vi "ChannelFlowUNDERGRAD.vi"() -> ()   [LabVIEW 2012]
uses:
  <vilib>/express/express shared/transition.llb/Dynamic To Waveform Array.vi
  <vilib>/express/express shared/transition.llb/Waveform Array To Dynamic.vi
  <vilib>/express/express arith-compare/Formula/Block/exnFormulaBlock how many pts in the wave.vi
  <vilib>/express/express shared/ex_Modify Signal Name.vi
  <vilib>/express/express analysis/Spectral/Block/exnSpectralBlock spectral measurements power poly.vi
  <vilib>/express/express analysis/Spectral/Block/exnSpectralBlock spectral measurements power DDT.vi
  <vilib>/Utility/file.llb/Write To Spreadsheet File (DBL).vi
  <vilib>/express/express arith-compare/Formula/XNode/ExpressFormulaBlockNode.xnode
  <vilib>/express/express analysis/Spectral/XNode/ExpressSpectralMeasurementsBlockNode.xnode
  <vilib>/Analysis/NI_AALBase.lvlib
panel:
  out "Tau(Pa)":dbl
  out "Voltage":dbl
  in  "Samples":i32=40000
  in  "Rate":i32=40000
  out "Waveform Graph":dynamicdata(graph)
  out "Filtered Signal":dynamicdata(graph)
  out "Frequency":dbl
  in  "Zero Voltage":dbl=-3.65209
  out "DC":dbl(knob) scale=0.0..10.0
  out "Delay Elapsed":dbl(slide) caption="Elapsed Time (s)" scale=0.0..1.0
  in  "Freq(Hz) 2":dbl min=0.0 max=60.0 step=1.0 format="%#_3g"
  in  "stop":bool
  in  "Delay Time (s)":dbl=5.0
  in  "Freq Increment":dbl=5.0 min=0.0 max=5.0 step=0.1
  in  "MaxF":dbl=55.0
  out "Flowm (gpm)":dbl
  in  "Freq(Hz)":dbl min=0.0 max=60.0 step=0.1 format="%#_3g"
  out "Waveform Chart":dynamicdata(graph)
  in  "Diaphragm":enum16{"-34", "-20"}(ring)
  out "Time left to save":dbl(slide) scale=0.0..1.0
  in  "Reset Graph":bool caption="Reset"
  out "Moody Diagram":cluster{"Y":dbl[], "Y":dbl[]}[](graph)
  in  "Start of run":dbl
  in  "Write to File?":bool
  in  "OK Button":bool
  in  "Sampling time":dbl=100.0
  in  "Sampling rate\n (0=10Hz)":dbl=100.0
  out "Viscosity (Pa s)":dbl format="%#_6e"
  out "Total Elapsed Time":dbl format="%#.0f"
  in  "stop 2":bool
  out "Bulk Velocity (m/s)":dbl
  in  "File Save Path":path=path "C:/Users/Picasso/Google Drive/Channel Data/SLIPS Data"
  out "Friction Factor":dbl
  out "Reynolds Number":dbl
  out "Density (kg/m^3)":dbl
  in  "Width (m)":dbl=0.1016
  in  "Length (m)":dbl=0.381
  in  "Half-height (m)":dbl=0.00195
  out "Temperature (C)":dbl
  in  "Flow Rate\n (Gpm)":dbl=15.6
  out "Pressure \nDifference (Pa)":dbl
  # "Inputs"
  # "Raw Data"
  # "Calculated Values"
  # "(DO NOT HIT RUN WITH THIS BLANK)"
  # "Pump Settings"
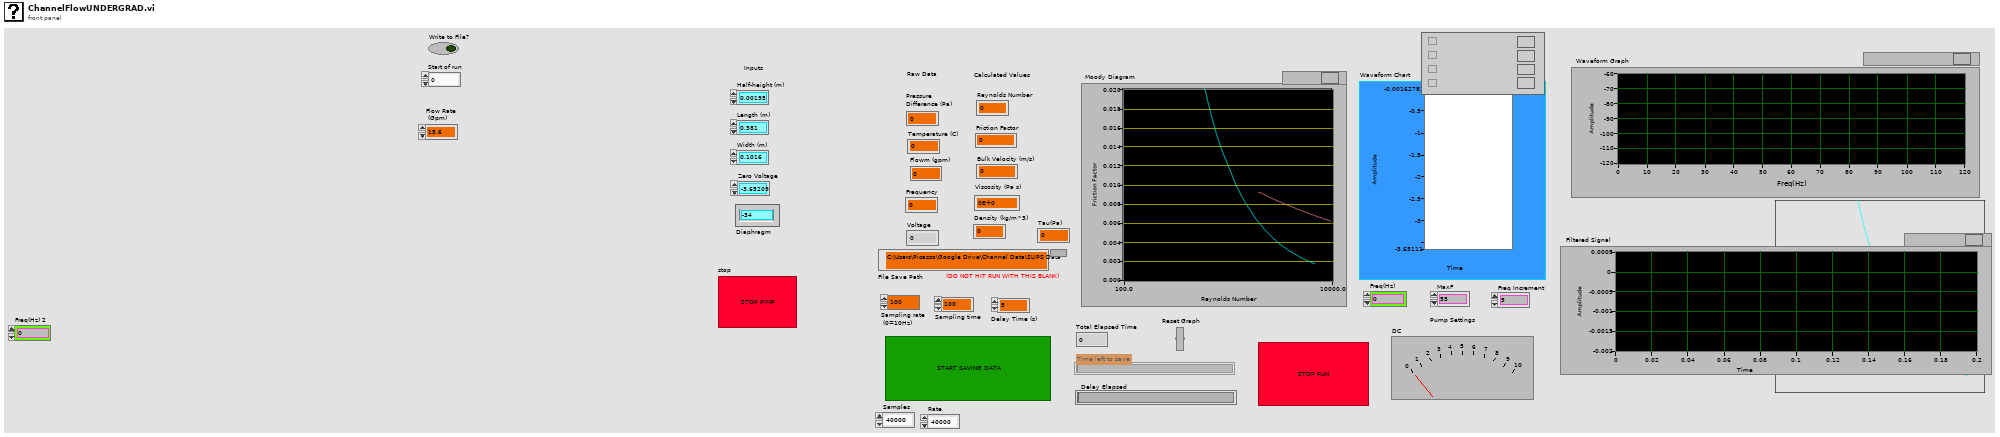
[diagram p1: front panel]
types:
  T1 = cluster{"averaging mode":u16, "weighting mode":u16, "number of averages":u32}
  T2 = cluster{"dB On (F)":bool, "unwrap phase (F)":bool, "convert to degree (F)":bool}
  T3 = enum8{"Enabled", "Disabled", "Disabled and Grayed Out"}
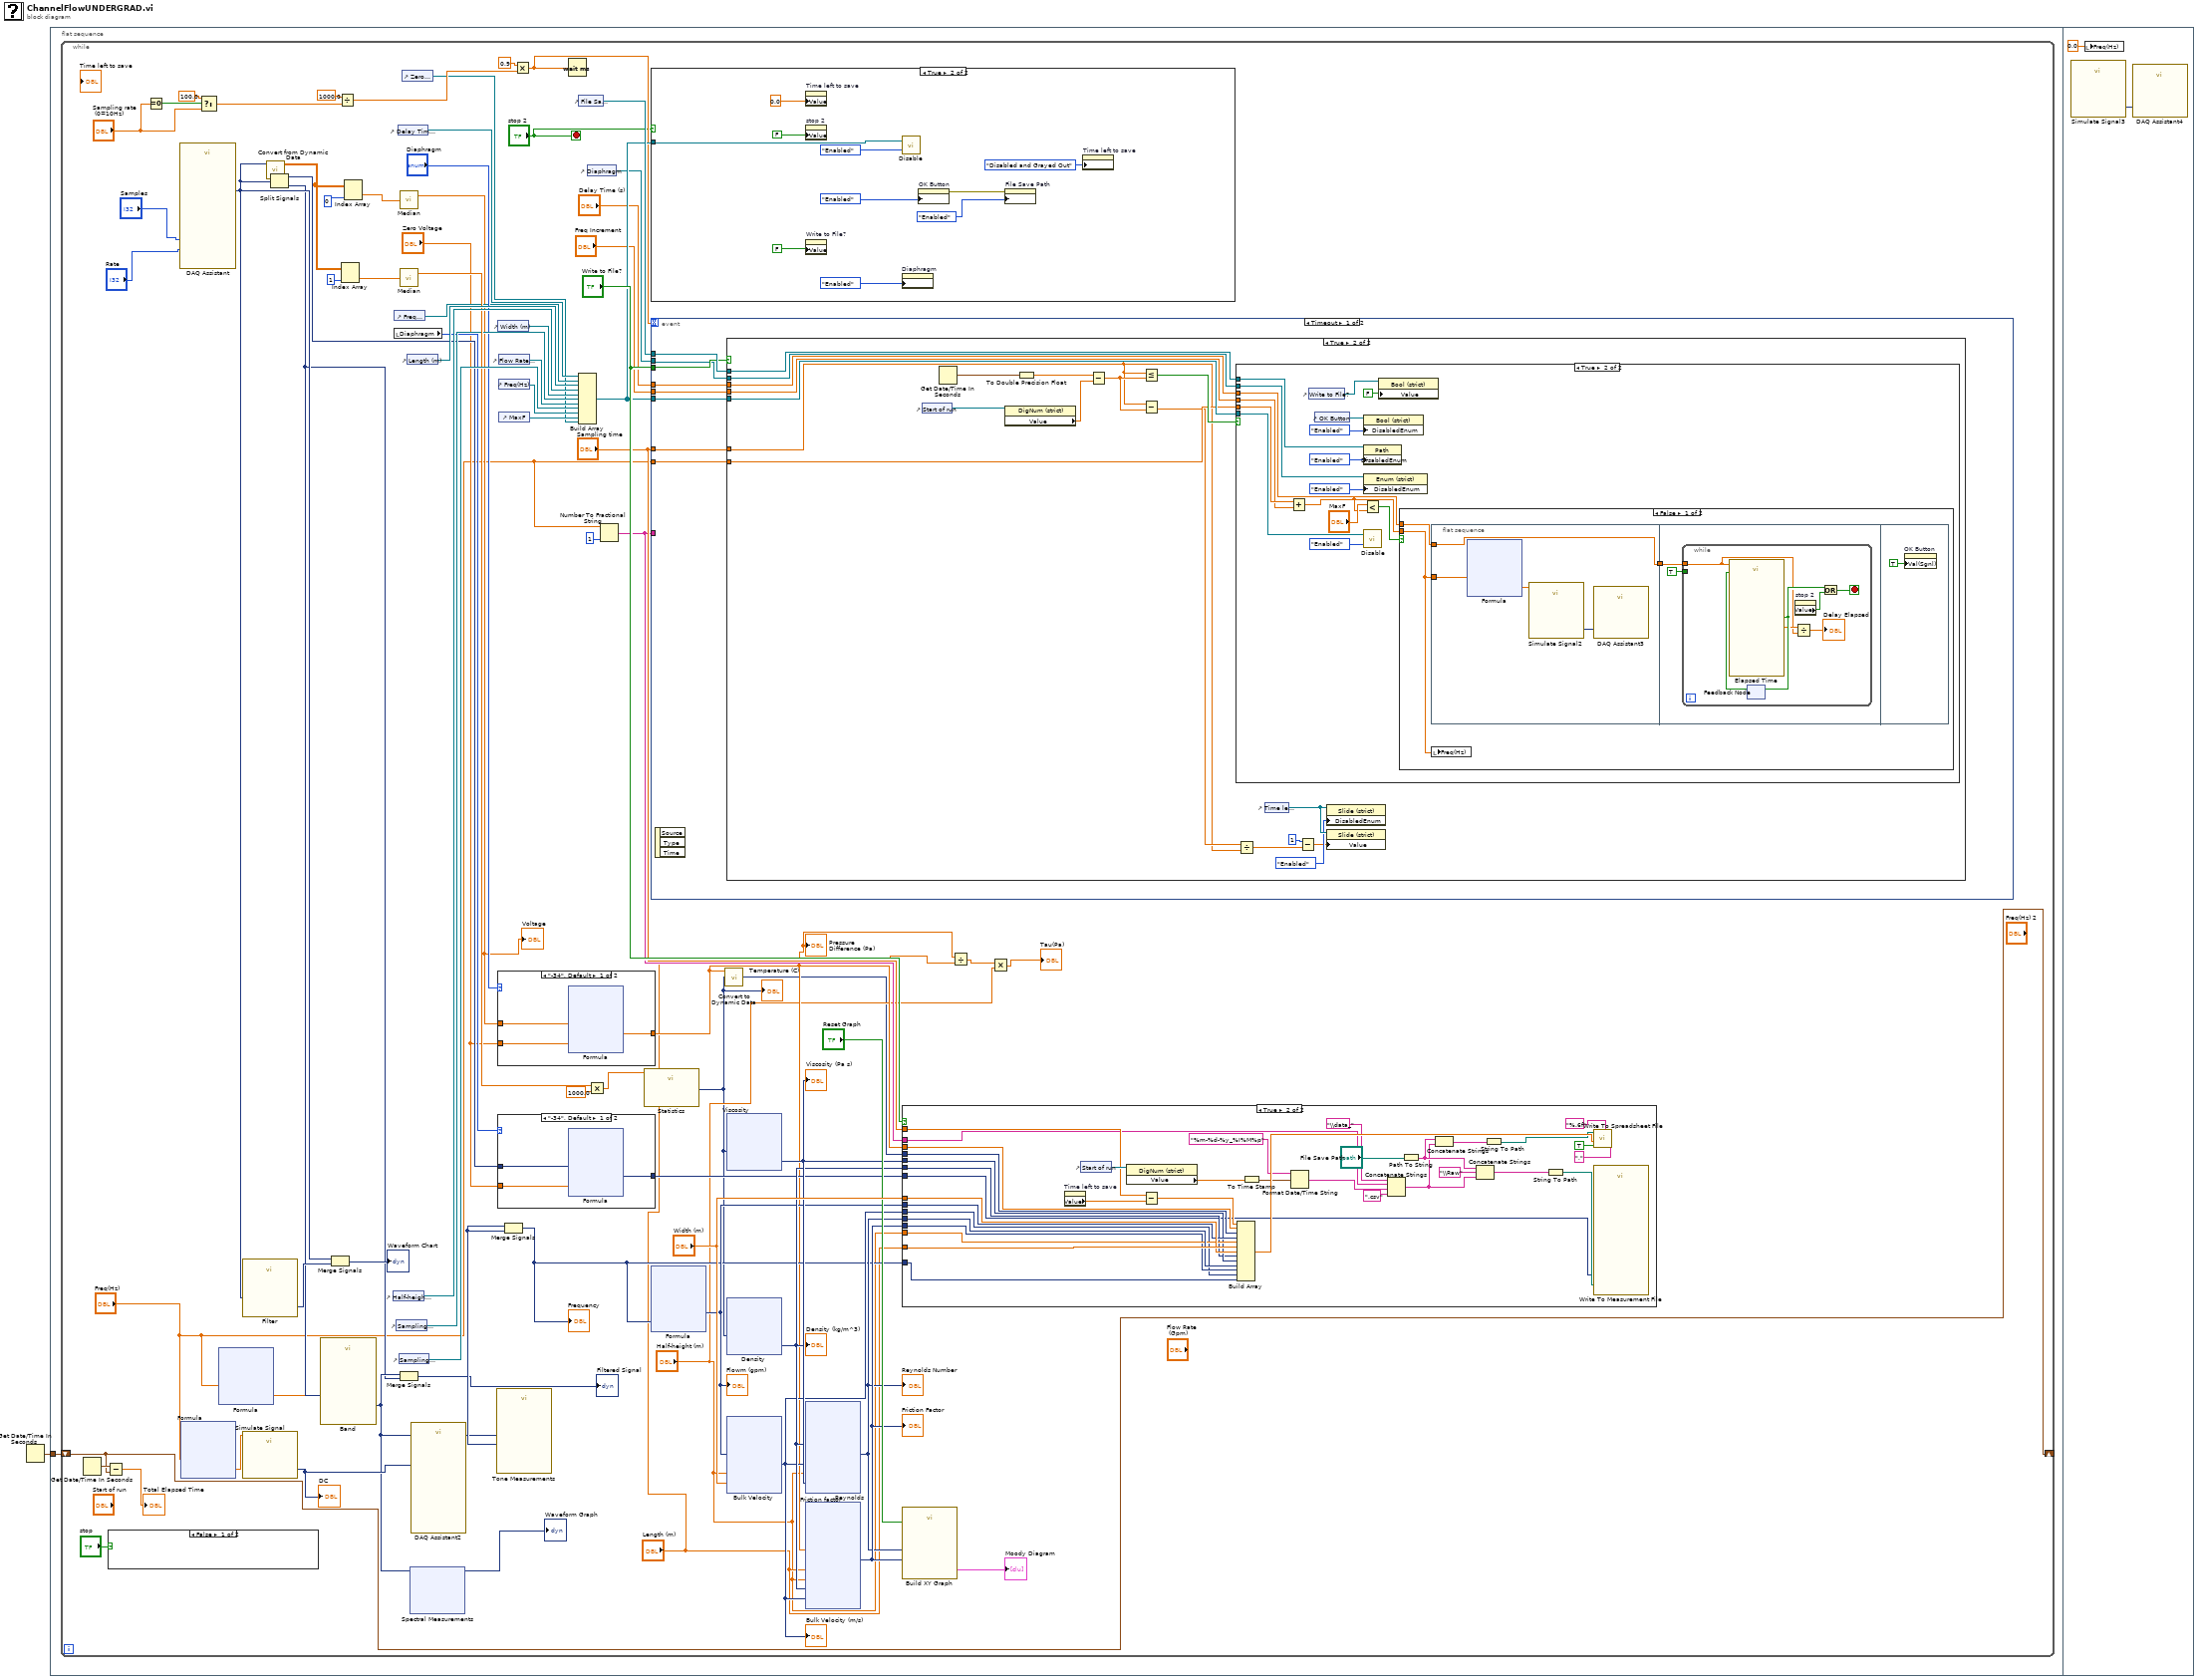
[diagram p0: block diagram]
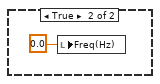
[diagram p2: hidden frame]
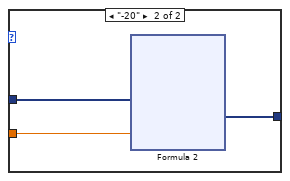
[diagram p3: hidden frame]
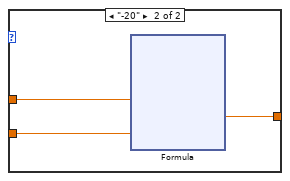
[diagram p4: hidden frame]
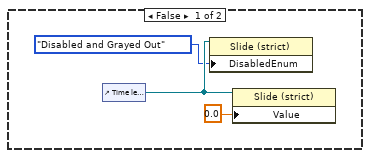
[diagram p7: hidden frame]
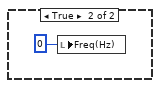
[diagram p9: hidden frame]
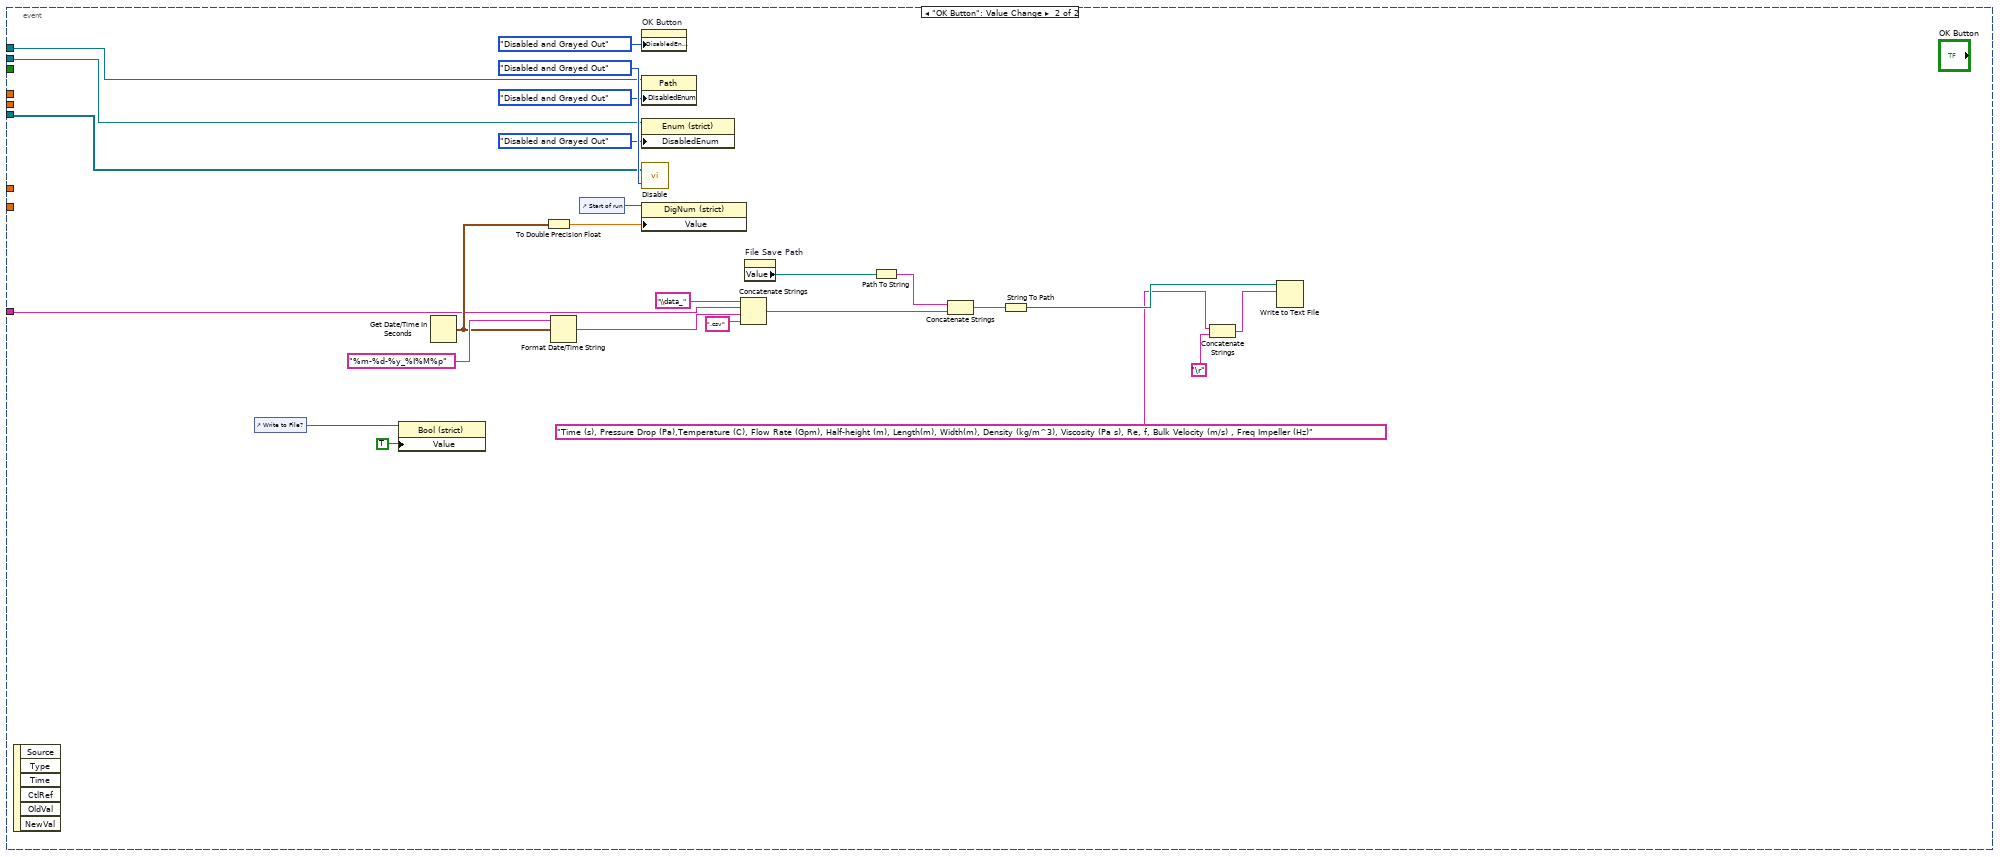
[diagram p10: hidden frame]
diagram:
  n1 = Get Date/Time In Seconds() -> (seconds since 1Jan1904=w1:timestamp)
  n2 = flat-sequence {
    tunnel: w1 -> [w2]
    frame #0 {
      n3 = while {
        shift-right: [w72] -> _
        shift-left: w2 -> [w72]
        stop <- "stop 2" stop-if-true
        n4 = Get Date/Time In Seconds() -> (seconds since 1Jan1904=w73:timestamp)
        n5 = Subtract(x=w73, y=w72) -> (x-y=→"Total Elapsed Time":dbl)
        n6 = case shown="False" "stop" {
          frame False {
          }
          frame True {
            n7 = local write "Freq(Hz)"(0.0) -> ()
          }
        }
        n8 = Equal To 0?(x="Sampling rate\n (0=10Hz)") -> (x = 0?=w69:bool)
        n9 = call "DAQ Assistant"("rate"="Rate", "number of samples"="Samples") -> ("data"=w34:dynamicdata)  [unwired: 15 in, 2 out]
        n10 = xnode "Formula"("X1"="Freq(Hz)") -> ("Result"=w38:dbl)  [unwired: 1 in, 1 out]
        n11 = Select(t=100.0, s=w69, f="Sampling rate\n (0=10Hz)") -> (s? t:f=w68:dbl)
        n12 = xnode "Formula"("X1"="Freq(Hz)") -> ("Result"=w10:dbl)  [unwired: 1 in, 1 out]
        n13 = call "Filter"("Signal"=w34) -> ("Filtered Signal"=w41:dynamicdata)  [unwired: 9 in, 1 out]
        n14 = call "Simulate Signal"("Offset"=w38) -> ("DC"=w37:dynamicdata)  [unwired: 13 in, 1 out]
        "DC" <- w37
        n15 = call "Convert from Dynamic Data"("Dynamic Data Type"=w34) -> ("Array"=w35:dbl[][])  [unwired: 3 in]
        n16 = Split Signals(w34) -> (w25:dynamicdata, w16:dynamicdata)  [unwired: 3 in, 1 out]
        n17 = call "Band"("Lower Cut-Off"=w10, "Signal"=w16) -> ("Filtered Signal"=w19:dynamicdata)  [unwired: 8 in, 1 out]
        n18 = Merge Signals(w34, w41) -> (→"Waveform Chart":dynamicdata)
        n19 = Divide(x=1000.0, y=w68) -> (x/y=w46:dbl)
        n20 = Index Array(array=w35, index (col)=1 ("index")) -> (element=w56:dbl[])  [unwired: 1 in]
        n21 = Index Array(array=w35, index (col)=0 ("index")) -> (element=w55:dbl[])  [unwired: 1 in]
        n22 = control-ref of="Half-height (m)"() -> (w79:refnum<vi>)
        n23 = control-ref of="Freq Increment"() -> (w29:refnum<vi>)
        n24 = local read "Diaphragm"() -> (w26:enum16{"-34", "-20"})
        n25 = control-ref of="Sampling time"() -> (w51:refnum<vi>)
        n26 = control-ref of="Delay Time (s)"() -> (w28:refnum<vi>)
        n27 = control-ref of="Sampling rate\n (0=10Hz)"() -> (w76:refnum<vi>)
        n28 = call <vilib>:"Median.vi"("X"=w55) -> ("median"=w12:dbl)  [unwired: 1 out]
        "Voltage" <- w12
        n29 = call <vilib>:"Median.vi"("X"=w56) -> ("median"=w53:dbl)  [unwired: 1 out]
        n30 = Merge Signals(w19, w16) -> (→"Filtered Signal":dynamicdata)
        n31 = control-ref of="Zero Voltage"() -> (w22:refnum<vi>)
        n32 = control-ref of="Length (m)"() -> (w78:refnum<vi>)
        n33 = xnode "Spectral Measurements"("Signals"=w19) -> ("Power Spectrum"=→"Waveform Graph":dynamicdata)  [unwired: 1 in, 1 out]
        n34 = call "DAQ Assistant2"("data"=w37) -> ()  [unwired: 17 in, 2 out]
        n35 = call "Tone Measurements"("Signals"=w19) -> ("Frequency"=w20:dynamicdata)  [unwired: 9 in, 1 out]
        n36 = control-ref of="Width (m)"() -> (w77:refnum<vi>)
        n37 = case shown="\"-34\", Default" "Diaphragm" {
          tunnel: w12 -> [w531 w544]
          tunnel: [w530 w543] -> w9
          tunnel: "Zero Voltage" -> [w529 w542]
          frame "-34", Default {
            n38 = xnode "Formula"("V"=w531, "X2"=w529) -> ("Result"=w530:dbl)  [unwired: 1 in, 1 out]
          }
          frame "-20" {
            n39 = xnode "Formula"("V"=w544, "X2"=w542) -> ("Result"=w543:dbl)  [unwired: 1 in, 1 out]
          }
        }
        "Pressure \nDifference (Pa)" <- w9
        n40 = case shown="\"-34\", Default" w26 {
          tunnel: [w100 w242] -> w27
          tunnel: w25 -> [w99 w241]
          tunnel: "Zero Voltage" -> [w98 w240]
          frame "-34", Default {
            n41 = xnode "Formula"("V"=w99, "X2"=w98) -> ("Result"=w100:dynamicdata)  [unwired: 1 in, 1 out]
          }
          frame "-20" {
            n42 = xnode "Formula 2"("V"=w241, "X2"=w240) -> ("Result"=w242:dynamicdata)  [unwired: 1 in, 1 out]
          }
        }
        n43 = control-ref of="Flow Rate\n (Gpm)"() -> (w50:refnum<vi>)
        n44 = control-ref of="Freq(Hz)"() -> (w36:refnum<vi>)
        n45 = control-ref of="MaxF"() -> (w32:refnum<vi>)
        n46 = Merge Signals(w20, w20) -> (w15:dynamicdata)
        "Frequency" <- w15
        n47 = Multiply(x=0.9, y=w46) -> (x*y=w43:dbl)
        n48 = Wait (ms)(milliseconds to wait=w43) -> ()  [unwired: 1 out]
        n49 = control-ref of="File Save Path"() -> (w75:refnum<vi>)
        n50 = Build Array(w28, w29, w78, w79, w77, w51, w50, w76, w36, w32, w22) -> (w62:refnum<vi>[])
        n51 = control-ref of="Diaphragm"() -> (w47:refnum<vi>)
        n52 = Multiply(x=w53, y=1000.0) -> (x*y=w4:dbl)
        n53 = Number To Fractional String(number="Freq(Hz)", precision (6)=1) -> (F-format string=w39:string)  [unwired: 2 in]
        n54 = call "Statistics"("Signals"=w4) -> ("Median"=w3:dynamicdata)  [unwired: 25 in, 1 out]
        "Temperature (C)" <- w3
        n55 = case shown="True" "stop 2" {
          tunnel: w62 -> [_ w842]
          frame False {
          }
          frame True {
            n56 = property on="Time left to save" class="Slide (strict)"("Value"=0.0 ("Time left to save")) -> ()  [unwired: 2 in, 2 out]
            n57 = property on="stop 2" class="Bool (strict)"("Value"=FALSE) -> ()  [unwired: 2 in, 2 out]
            n58 = property on="Write to File?" class="Bool (strict)"("Value"=FALSE ("Write to File?")) -> ()  [unwired: 2 in, 2 out]
            n59 = call "Disable.vi"("Disabled"=T3."Enabled", "Array"=w842) -> ()  [unwired: 1 in]
            n60 = property on="Diaphragm" class="Enum (strict)"("DisabledEnum"=T3."Enabled" ("Disabled")) -> ()  [unwired: 2 in, 2 out]
            n61 = property on="OK Button" class="Bool (strict)"("DisabledEnum"=T3."Enabled" ("Disabled")) -> (error out=w839:errorcluster)  [unwired: 2 in, 1 out]
            n62 = property on="File Save Path" class="Path"(error in=w839, "DisabledEnum"=T3."Enabled" ("Disabled")) -> ()  [unwired: 1 in, 2 out]
            n63 = property on="Time left to save" class="Slide (strict)"("DisabledEnum"=T3."Disabled and Grayed Out" ("Disabled")) -> ()  [unwired: 2 in, 2 out]
          }
        }
        n64 = event shown="[0] Timeout" {
          selector: _ -> [_ _]
          dyn-events: _ -> [_ _]
          timeout: w43 -> [_ _]
          tunnel: w62 -> [w1302 w1389]
          tunnel: w75 -> [w1301 w1388]
          tunnel: "Sampling time" -> [w1303 _]
          tunnel: "Write to File?" -> [w1300 _]
          tunnel: w47 -> [w1299 w1374]
          tunnel: w39 -> [_ w1371]
          tunnel: "Freq(Hz)" -> [w1298 _]
          tunnel: "Freq Increment" -> [w1297 _]
          tunnel: "Delay Time (s)" -> [w1296 _]
          event Timeout {
            n65 = event-data() -> ()  [unwired: 1 in, 3 out]
            n66 = case shown="True" w1300 {
              tunnel: w1303 -> [_ w1310]
              tunnel: w1302 -> [_ w1323]
              tunnel: w1301 -> [_ w1322]
              tunnel: w1299 -> [_ w1318]
              tunnel: w1298 -> [_ w1314]
              tunnel: w1297 -> [_ w1313]
              tunnel: w1296 -> [_ w1312]
              frame False {
                n67 = control-ref of="Time left to save"() -> (w1305:refnum<vi>)
                n68 = property class="Slide (strict)"(reference=w1305, "DisabledEnum"=T3."Disabled and Grayed Out" ("Disabled")) -> ()  [unwired: 1 in, 2 out]
                n69 = property class="Slide (strict)"(reference=w1305, "Value"=0.0) -> ()  [unwired: 1 in, 2 out]
              }
              frame True {
                n70 = control-ref of="Start of run"() -> (w1325:refnum<vi>)
                n71 = Get Date/Time In Seconds() -> (seconds since 1Jan1904=w1316:timestamp)
                n72 = property class="DigNum (strict)"(reference=w1325) -> ("Value"=w1324:dbl)  [unwired: 1 in, 2 out]
                n73 = To Double Precision Float(number=w1316) -> (double precision float=w1315:dbl)
                n74 = Subtract(x=w1315, y=w1324) -> (x-y=w1317:dbl)
                n75 = Less Or Equal?(x=w1310, y=w1317) -> (x <= y?=w1321:bool)
                n76 = Subtract(x=w1310, y=w1317) -> (x-y=w1311:dbl)
                n77 = case shown="True" w1321 {
                  tunnel: w1323 -> [_ w1338]
                  tunnel: w1322 -> [_ w1337]
                  tunnel: w1318 -> [_ w1332]
                  tunnel: w1314 -> [_ w1329]
                  tunnel: w1313 -> [_ w1327]
                  tunnel: w1312 -> [_ w1326]
                  frame False {
                  }
                  frame True {
                    n78 = Add(x=w1329, y=w1327) -> (x+y=w1328:dbl)
                    n79 = control-ref of="Write to File?"() -> (w1335:refnum<vi>)
                    n80 = control-ref of="OK Button"() -> (w1336:refnum<vi>)
                    n81 = property class="Bool (strict)"(reference=w1336, "DisabledEnum"=T3."Enabled" ("Disabled")) -> ()  [unwired: 1 in, 2 out]
                    n82 = property class="Path"(reference=w1337, "DisabledEnum"=T3."Enabled" ("Disabled")) -> ()  [unwired: 1 in, 2 out]
                    n83 = property class="Enum (strict)"(reference=w1332, "DisabledEnum"=T3."Enabled" ("Disabled")) -> ()  [unwired: 1 in, 2 out]
                    n84 = Less?(x="MaxF", y=w1328) -> (x < y?=w1330:bool)
                    n85 = call "Disable.vi"("Disabled"=T3."Enabled", "Array"=w1338) -> ()  [unwired: 1 in]
                    n86 = property class="Bool (strict)"(reference=w1335, "Value"=FALSE) -> ()  [unwired: 1 in, 2 out]
                    n87 = case shown="False" w1330 {
                      tunnel: w1328 -> [w1344 _]
                      tunnel: w1326 -> [w1343 _]
                      frame False {
                        n88 = flat-sequence {
                          tunnel: w1344 -> [w1346]
                          tunnel: w1343 -> [w1345]
                          tunnel: [w1345] -> w1342
                          tunnel: w1342 -> [w1358]
                          frame #0 {
                            n89 = xnode "Formula"("X1"=w1346) -> ("Result"=w1348:dbl)  [unwired: 1 in, 1 out]
                            n90 = call "Simulate Signal2"("Offset"=w1348) -> ("DC"=w1347:dynamicdata)  [unwired: 13 in, 1 out]
                            n91 = call "DAQ Assistant3"("data"=w1347) -> ()  [unwired: 17 in, 2 out]
                          }
                          frame #1 {
                            n92 = while {
                              tunnel: w1358 -> [w1360]
                              tunnel: TRUE -> [_]
                              stop <- w1362 stop-if-true
                              n93 = feedback #1() -> (w1365:bool)  [unwired: 1 in]
                              n94 = call "Elapsed Time"("Time Target (s)"=w1360, "Reset"=w1365) -> ("Elapsed Time (s)"=w1361:dbl, "Time has Elapsed"=w1363:bool)  [unwired: 10 in, 6 out]
                              n95 = feedback-in #1(w1363) -> ()
                              n96 = property on="stop 2" class="Bool (strict)"() -> ("Value"=w1364:bool)  [unwired: 2 in, 2 out]
                              n97 = Divide(x=w1361, y=w1360) -> (x/y=→"Delay Elapsed":dbl)
                              n98 = Or(x=w1363, y=w1364) -> (x .or. y?=w1362:bool)
                            }
                          }
                          frame #2 {
                            n99 = property on="OK Button" class="Bool (strict)"("Val(Sgnl)"=TRUE) -> ()  [unwired: 2 in, 2 out]
                          }
                        }
                        n100 = local write "Freq(Hz)"(w1344) -> ()
                      }
                      frame True {
                        n101 = local write "Freq(Hz)"(0) -> ()
                      }
                    }
                  }
                }
                n102 = Divide(x=w1311, y=w1310) -> (x/y=w1309:dbl)
                n103 = control-ref of="Time left to save"() -> (w1320:refnum<vi>)
                n104 = Subtract(x=1, y=w1309) -> (x-y=w1307:dbl)
                n105 = property class="Slide (strict)"(reference=w1320, "DisabledEnum"=T3."Enabled" ("Disabled")) -> ()  [unwired: 1 in, 2 out]
                n106 = property class="Slide (strict)"(reference=w1320, "Value"=w1307) -> ()  [unwired: 1 in, 2 out]
              }
            }
          }
          event "OK Button": Value Change {
            n107 = event-data() -> ()  [unwired: 1 in, 6 out]
            n108 = control-ref of="Write to File?"() -> (w1387:refnum<vi>)
            n109 = property class="Bool (strict)"(reference=w1387, "Value"=TRUE) -> ()  [unwired: 1 in, 2 out]
            n110 = Get Date/Time In Seconds() -> (seconds since 1Jan1904=w1377:timestamp)
            n111 = To Double Precision Float(number=w1377) -> (double precision float=w1384:dbl)
            n112 = Format Date/Time String(time format string (%c)="%m-%d-%y_%I%M%p", seconds (now)=w1377) -> (date/time string=w1372:string)  [unwired: 1 in]
            n113 = control-ref of="Start of run"() -> (w1385:refnum<vi>)
            n114 = property on="OK Button" class="Bool (strict)"("DisabledEnum"=T3."Disabled and Grayed Out" ("Disabled")) -> ()  [unwired: 2 in, 2 out]
            n115 = property class="Path"(reference=w1388, "DisabledEnum"=T3."Disabled and Grayed Out" ("Disabled")) -> ()  [unwired: 1 in, 2 out]
            n116 = property class="Enum (strict)"(reference=w1374, "DisabledEnum"=T3."Disabled and Grayed Out" ("Disabled")) -> ()  [unwired: 1 in, 2 out]
            n117 = call "Disable.vi"("Disabled"=T3."Disabled and Grayed Out", "Array"=w1389) -> ()  [unwired: 1 in]
            n118 = property class="DigNum (strict)"(reference=w1385, "Value"=w1384) -> ()  [unwired: 1 in, 2 out]
            n119 = Concatenate Strings("\\data_", w1371, w1372, ".csv" ("string")) -> (w1379:string)
            n120 = property on="File Save Path" class="Path"() -> ("Value"=w1378:path)  [unwired: 2 in, 2 out]
            n121 = Path To String(path=w1378) -> (string=w1380:string)
            n122 = Concatenate Strings(w1380, w1379) -> (w1381:string)
            n123 = String To Path(string=w1381) -> (path=w1376:path)
            n124 = Concatenate Strings("Time (s), Pressure Drop (Pa),Temperature (C), Flow Rate (Gpm), Half-height (m), Length(m), Width(m), Density (kg/m^3), Viscosity (Pa s), Re, f, Bulk Velocity (m/s) , Freq Impeller (Hz)" ("text"), "\r") -> (w1368:string)
            n125 = Write to Text File(file (use dialog)=w1376, text=w1368) -> ()  [unwired: 2 in, 3 out]
          }
        }
        n126 = xnode "Formula"("X1"=w15) -> ("Result"=w23:dynamicdata)  [unwired: 1 in, 1 out]
        "Flowm (gpm)" <- w23
        n127 = call "Convert to Dynamic Data"("Double"=w9) -> ()  [unwired: 3 in, 1 out]
        n128 = xnode "Viscosity"("T"=w3) -> ("Result"=w60:dynamicdata)  [unwired: 1 in, 1 out]
        "Viscosity (Pa s)" <- w60
        n129 = xnode "Density"("T"=w3) -> ("Result"=w59:dynamicdata)  [unwired: 1 in, 1 out]
        "Density (kg/m^3)" <- w59
        n130 = xnode "Bulk Velocity"("Q"=w23, "h"="Half-height (m)", "w"="Width (m)") -> ("Result"=w49:dynamicdata)  [unwired: 1 in, 1 out]
        "Bulk Velocity (m/s)" <- w49
        n131 = xnode "Reynolds"("r"=w59, "U"=w49, "h"="Half-height (m)", "m"=w60) -> ("Result"=w52:dynamicdata)  [unwired: 1 in, 1 out]
        "Reynolds Number" <- w52
        n132 = xnode "Friction factor"("P"=w9, "L"="Length (m)", "h"="Half-height (m)", "r"=w59, "U"=w49) -> ("Result"=w61:dynamicdata)  [unwired: 1 in, 1 out]
        "Friction Factor" <- w61
        n133 = case shown="True" "Write to File?" {
          tunnel: w23 -> [_ w872]
          tunnel: "Half-height (m)" -> [_ w865]
          tunnel: "Length (m)" -> [_ w878]
          tunnel: "Width (m)" -> [_ w877]
          tunnel: w52 -> [_ w876]
          tunnel: w61 -> [_ w864]
          tunnel: w60 -> [_ w863]
          tunnel: w59 -> [_ w862]
          tunnel: w9 -> [_ w860]
          tunnel: w3 -> [_ w859]
          tunnel: w49 -> [_ w858]
          tunnel: "Sampling time" -> [_ w854]
          tunnel: w39 -> [_ w851]
          tunnel: w27 -> [_ w844]
          tunnel: w15 -> [_ w843]
          frame False {
          }
          frame True {
            n134 = property on="Time left to save" class="Slide (strict)"() -> ("Value"=w856:dbl)  [unwired: 2 in, 2 out]
            n135 = control-ref of="Start of run"() -> (w870:refnum<vi>)
            n136 = property class="DigNum (strict)"(reference=w870) -> ("Value"=w869:dbl)  [unwired: 1 in, 2 out]
            n137 = Subtract(x=w854, y=w856) -> (x-y=w855:dbl)
            n138 = Build Array(w855, w860, w859, w872, w865, w878, w877, w862, w863, w876, w864, w858, w843) -> (w875:dbl[])
            n139 = To Time Stamp(1:w869) -> (0:w868:timestamp)
            n140 = Format Date/Time String(time format string (%c)="%m-%d-%y_%I%M%p", seconds (now)=w868) -> (date/time string=w852:string)  [unwired: 1 in]
            n141 = Concatenate Strings("\\data_", w851, w852, ".csv" ("string")) -> (w845:string)
            n142 = Path To String(path="File Save Path") -> (string=w846:string)
            n143 = Concatenate Strings(w846, w845) -> (w848:string)
            n144 = Concatenate Strings(w846, "\\Raw", w845) -> (w850:string)
            n145 = String To Path(string=w848) -> (path=w866:path)
            n146 = String To Path(string=w850) -> (path=w849:path)
            n147 = call-poly <vilib>:"Write To Spreadsheet File.vi"("delimiter (\\t)"="," ("delimiter (\\t)"), "format (%.3f)"="%.6f", "append to file? (new file:F)"=TRUE, "1D data"=w875, "file path (dialog if empty)"=w866) -> ()  [unwired: 3 in, 1 out]
            n148 = call "Write To Measurement File"("Signals"=w844, "Filename"=w849) -> ()  [unwired: 15 in, 3 out]
          }
        }
        n149 = call "Build XY Graph"("Reset"="Reset Graph", "Y Input"=w61, "X Input"=w52) -> ("XY Graph"=→"Moody Diagram":cluster{"X":dbl[], "Y":dbl[]}[])  [unwired: 7 in, 1 out]
        n150 = Divide(x=w9, y="Length (m)") -> (x/y=w7:dbl)
        n151 = Multiply(x=w7, y="Half-height (m)") -> (x*y=→"Tau(Pa)":dbl)
      }
    }
    frame #1 {
      n152 = call "Simulate Signal3"() -> ("DC"=w1394:dynamicdata)  [unwired: 14 in, 1 out]
      n153 = local write "Freq(Hz)"(0.0) -> ()
      n154 = call "DAQ Assistant4"("data"=w1394) -> ()  [unwired: 17 in, 2 out]
    }
  }
